vi "Zapamietaj LogAdr.vi"(7 "Akcja (GET)":T1, 11 "Directory in":path) -> (3 "Directory out":path)   [LabVIEW 2014]
doc: "Zapamietuje w zmiennej FGV adres do logowania b³êdów"
uses:
  Kontrolki/FVGs/FVG akcje podstawowa.ctl
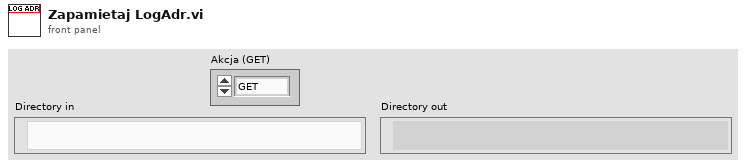
[diagram p1: front panel]
types:
  T1 = typedef "FVG akcje podstawowa.ctl" = enum16{"GET", "SET"}
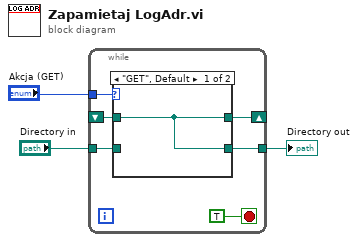
[diagram p0: block diagram]
diagram:
  n1 = while {
    tunnel: "Akcja (GET)" -> [w8]
    tunnel: "Directory in" -> [w7]
    tunnel: [w6] -> w1
    shift-right: [w5] -> _
    shift-left: _ -> [w4]
    stop <- TRUE stop-if-true
    n2 = case shown="\"GET\", Default" w8 {
      tunnel: w7 -> [_ w11]
      tunnel: [w10 w11] -> w6
      tunnel: [w10 w11] -> w5
      tunnel: w4 -> [w10 _]
      frame "GET", Default {
      }
      frame "SET" {
      }
    }
  }
  "Directory out" <- w1
